vi "AIM664 Receive Data.vi"() -> ()   [LabVIEW 2020]
uses:
  src/AIM664LV.lvlib
panel:
  out "error out":errorcluster
  out "QueueIdOut 2":u32=664064
  out "GlobMonSize 2":u32=2153143691
  out "QueueIdOut":u32=664064
  out "GlobMonSize":u32=2153143691
  in  "Strobe":u32(ring) items=["FDX_MON_STROBE_DIS", "FDX_MON_STROBE_STOP", "FDX_MON_STROBE_START"]
  in  "TriggerPosition":u32
  in  "CaptureMode":u32(ring) items=["FDX_MON_SINGLE ", "FDX_MON_CONTINUOUS", "FDX_MON_SELECTIVE", "FDX_MON_RECORDING", "FDX_MON_REROS", "FDX_MON_HMU"]
  out "ResourceInfo 2":T1 {"PortMode" items=[" FDX_SINGLE", "FDX_REDUNDANT"]}
  out "ResourceInfo":T1 {"PortMode" items=[" FDX_SINGLE", "FDX_REDUNDANT"]}
  in  "Input Cluster 2":T2={"QueueCtrl"=1, "QueueId"=0, "RecordingFileName"="", "MaxFileSize"=0} {"QueueCtrl" items=["FDX_MON_QUEUE_CREATE", "FDX_MON_QUEUE_DELETE"]}
  in  "Stop":bool
  out "Output Cluste":T3={"EntryRead"=1, "BytesRead"=128, "Synchronized"=0, "ReadBuffer"=[192, 16, 128, 0, 192, 17, 128, 0, 0, 0, 0, 0, 0, 0, 0, 0, 60, 0, 0, 0, 64, 64, 0, 48, 84, 0, 128, 0, 104, 8, 0, 0, 33, 75, 42, 162, 3, 0, 0, 0, 0, 60, 2, 0, 0, 1, 33, 32, 8, 0, 69, 0, 0, 45, 0, 0, 64, 0, 1, 17, 109, 162, 10, 1, 33, 1, 224, 224, 0, 60, 0, 24, 0, 23, 0, 25, 0, 0, 65, 66, 67, 68, 69, 70, 71, 72, 73, 74, 75, 76, 77, 78, 79, 80, 81, 84, 0, 5, 0, 5, 0, 5, 0, 5, 0, 5, 0, 5, 0, 5, 0, 5, 0, 5, 0, 5, 0, 5, 0, 5, 0, 5, 0, 5, 0, 5, 0, 5, 0, 0, 0, 0, 0, 0, 0, 0, 0, 0, 0, 0, 0, 0, 0, 0, 0, 0, 0, 0, 0, 0, 0, 0, 0, 0, 0, 0, 0, 0, 0, 0, 0, 0, 0, 0, 0, 0, 0, 0, 0, 0, 0, 0, 0, 0, 0, 0, 0, 0, 0, 0, 0, 0, 0, 0, 0, 0, 0, 0, 0, 0, 0, 0, 0, 0, 0, 0, 0, 0, 0, 0, 0, 0, 0, 0, 0, 0, 0, 0, 0, 0, 0, 0, 0, 0, 0, 0, 0, 0, 0, 0, 0, 0, 0, 0, 0, 0, 0, 0, 0, 0, 0, 0, 0, 0, 0, 0, 0, 0, 0, 0, 0, 0, 0, 0, 0, 0, 0, 0, 0, 0, 0, 0, 0, 0, 0, 0, 0, 0, 0, 0, 0, 0, 0, 0, 0, 0, 0, 0, 0, 0, 0, 0, 0, 0, 0, 0, 0, 0, 0, 0, 0, 0, 0, 0, 0, 0, 0, 0, 0, 0, 0, 0, 0, 0, 0, 0, 0, 0, 0, 0, 0, 0, 0, 0, 0, 0, 0, 0, 0, 0, 0, 0, 0, 0, 0, 0, 0, 0, 0, 0, 0, 0, 0, 0, 0, 0, 0, 0, 0, 0, 0, 0, 0, 0, 0, 0, 0, 0, 0, 0, 0, 0, 0, 0, 0, 0, 0, 0, 0, 0, 0, 0, 0, 0, 0, 0, 0, 0, 0, 0, 0, 0, 0, 0, 0, 0, 0, 0, 0, 0, 0, 0, 0, 0, 0, 0, 0, 0, 0, 0, 0, 0, 0, 0, 0, 0, 0, 0, 0, 0, 0, 0, 0, 0, 0, 0, 0, 0, 0, 0, 0, 0, 0, 0, 0, 0, 0, 0, 0, 0, 0, 0, 0, 0, 0, 0, 0, 0, 0, 0, 0, 0, 0, 0, 0, 0, 0, 0, 0, 0, 0, 0, 0, 0, 0, 0, 0, 0, 0, 0, 0, 0, 0, 0, 0, 0, 0, 0, 0, 0, 0, 0, 0, 0, 0, 0, 0, 0, 0, 0, 0, 0, 0, 0, 0, 0, 0, 0, 0, 0, 0, 0, 0, 0, 0, 0, 0, 0, 0, 0, 0, 0, 0, 0, 0, 0, 0, 0, 0, 0, 0, 0, 0, 0, 0, 0, 0, 0, 0, 0, 0, 0, 0, 0, 0, 0, 0, 0, 0, 0, 0, 0, 0, 0, 0, 0, 0, 0, 0, 0, 0, 0, 0, 0, 0, 0, 0, 0, 0, 0, 0, 0, 0, 0, 0, 0, 0, 0, 0, 0, 0, 0, 0, 0, 0, 0, 0, 0, 0, 0, 0, 0, 0, 0, 0, 0, 0, 0, 0, 0, 0, 0, 0, 0, 0, 0, 0, 0, 0, 0, 0, 0, 0, 0, 0, 0, 0, 0, 0, 0, 0, 0, 0, 0, 0, 0, 0, 0, 0, 0, 0, 0, 0, 0, 0, 0, 0, 0, 0, 0, 0, 0, 0, 0, 0, 0, 0, 0, 0, 0, 0, 0, 0, 0, 0, 0, 0, 0, 0, 0, 0, 0, 0, 0, 0, 0, 0, 0, 0, 0, 0, 0, 0, 0, 0, 0, 0, 0, 0, 0, 0, 0, 0, 0, 0, 0, 0, 0, 0, 0, 0, 0, 0, 0, 0, 0, 0, 0, 0, 0, 0, 0, 0, 0, 0, 0, 0, 0, 0, 0, 0, 0, 0, 0, 0, 0, 0, 0, 0, 0, 0, 0, 0, 0, 0, 0, 0, 0, 0, 0, 0, 0, 0, 0, 0, 0, 0, 0, 0, 0, 0, 0, 0, 0, 0, 0, 0, 0, 0, 0, 0, 0, 0, 0, 0, 0, 0, 0, 0, 0, 0, 0, 0, 0, 0, 0, 0, 0, 0, 0, 0, 0, 0, 0, 0, 0, 0, 0, 0, 0, 0, 0, 0, 0, 0, 0, 0, 0, 0, 0, 0, 0, 0, 0, 0, 0, 0, 0, 0, 0, 0, 0, 0, 0, 0, 0, 0, 0, 0, 0, 0, 0, 0, 0, 0, 0, 0, 0, 0, 0, 0, 0, 0, 0, 0, 0, 0, 0, 0, 0, 0, 0, 0, 0, 0, 0, 0, 0, 0, 0, 0, 0, 0, 0, 0, 0, 0, 0, 0, 0, 0, 0, 0, 0, 0, 0, 0, 0, 0, 0, 0, 0, 0, 0, 0, 0, 0, 0, 0, 0, 0, 0, 0, 0, 0, 0, 0, 0, 0, 0, 0, 0, 0, 0, 0, 0, 0, 0, 0, 0, 0, 0, 0, 0, 0, 0, 0, 0, 0, 0, 0, 0, 0, 0, 0, 0, 0, 0, 0, 0, 0, 0, 0, 0, 0, 0, 0, 0, 0, 0, 0, 0, 0, 0, 0, 0, 0, 0, 0, 0, 0, 0, 0, 0, 0, 0, 0, 0, 0, 0, 0, 0, 0, 0, 0, 0, 0, 0, 0, 0, 0, 0, 0, 0, 0, 0, 0, 0, 0, 0, 0, 0, 0, 0, 0, 0, 0, 0, 0, 0, 0, 0, 0, 0, 0, 0, 0, 0, 0, 0, 0, 0, 0, 0, 0, 0, 0, 0, 0, 0, 0, 0, 0, 0, 0, 0, 0, 0, 0, 0, 0, 0, 0, 0, 0, 0, 0, 0, 0, 0, 0, 0, 0, 0, 0, 0, 0, 0, 0, 0, 0, 0, 0, 0, 0, 0, 0, 0, 0, 0, 0, 0, 0, 0, 0, 0, 0, 0, 0, 0, 0, 0, 0, 0, 0, 0, 0, 0, 0, 0, 0, 0, 0, 0, 0, 0, 0, 0, 0, 0, 0, 0, 0, 0, 0, 0, 0, 0, 0, 0, 0, 0, 0, 0, 0, 0, 0, 0, 0, 0, 0, 0, 0, 0, 0, 0, 0, 0, 0, 0, 0, 0, 0, 0, 0, 0, 0, 0, 0, 0, 0, 0, 0, 0, 0, 0, 0, 0, 0, 0, 0, 0, 0, 0, 0, 0, 0, 0, 0, 0, 0, 0, 0, 0, 0, 0, 0, 0, 0, 0, 0, 0, 0, 0, 0, 0, 0, 0, 0, 0, 0, 0, 0, 0, 0, 0, 0, 0, 0, 0, 0, 0, 0, 0, 0, 0, 0, 0, 0, 0, 0, 0, 0, 0, 0, 0, 0, 0, 0, 0, 0, 0, 0, 0, 0, 0, 0, 0, 0, 0, 0, 0, 0, 0, 0, 0, 0, 0, 0, 0, 0, 0, 0, 0, 0, 0, 0, 0, 0, 0, 0, 0, 0, 0, 0, 0, 0, 0, 0, 0, 0, 0, 0, 0, 0, 0, 0, 0, 0, 0, 0, 0, 0, 0, 0, 0, 0, 0, 0, 0, 0, 0, 0, 0, 0, 0, 0, 0, 0, 0, 0, 0, 0, 0, 0, 0, 0, 0, 0, 0, 0, 0, 0, 0, 0, 0, 0, 0, 0, 0, 0, 0, 0, 0, 0, 0, 0, 0, 0, 0, 0, 0, 0, 0, 0, 0, 0, 0, 0, 0, 0, 0, 0, 0, 0, 0, 0, 0, 0, 0, 0, 0, 0, 0, 0, 0, 0, 0, 0, 0, 0, 0, 0, 0, 0, 0, 0, 0, 0, 0, 0, 0, 0, 0, 0, 0, 0, 0, 0, 0, 0, 0, 0, 0, 0, 0, 0, 0, 0, 0, 0, 0, 0, 0, 0, 0, 0, 0, 0, 0, 0, 0, 0, 0, 0, 0, 0, 0, 0, 0, 0, 0, 0, 0, 0, 0, 0, 0, 0, 0, 0, 0, 0, 0, 0, 0, 0, 0, 0, 0, 0, 0, 0, 0, 0, 0, 0, 0, 0, 0, 0, 0, 0, 0, 0, 0, 0, 0, 0, 0, 0, 0, 0, 0, 0, 0, 0, 0, 0, 0, 0, 0, 0, 0, 0, 0, 0, 0, 0, 0, 0, 0, 0, 0, 0, 0, 0, 0, 0, 0, 0, 0, 0, 0, 0, 0, 0, 0, 0, 0, 0, 0, 0, 0, 0, 0, 0, 0, 0, 0, 0, 0, 0, 0, 0, 0, 0, 0, 0, 0, 0, 0, 0, 0, 0, 0, 0, 0, 0, 0, 0, 0, 0, 0, 0, 0, 0, 0, 0, 0, 0, 0, 0, 0, 0, 0, 0, 0, 0, 0, 0, 0, 0, 0, 0, 0, 0, 0, 0, 0, 0, 0, 0, 0, 0, 0, 0, 0, 0, 0, 0, 0, 0, 0, 0, 0, 0, 0, 0, 0, 0, 0, 0, 0, 0, 0, 0, 0, 0, 0, 0, 0, 0, 0, 0, 0, 0, 0, 0, 0, 0, 0, 0, 0, 0, 0, 0, 0, 0, 0, 0, 0, 0, 0, 0, 0, 0, 0, 0, 0, 0, 0, 0, 0, 0, 0, 0, 0, 0, 0, 0, 0, 0, 0, 0, 0, 0, 0, 0, 0, 0, 0, 0, 0, 0, 0, 0, 0, 0, 0, 0, 0, 0, 0, 0, 0, 0, 0, 0, 0, 0, 0, 0, 0, 0, 0, 0, 0, 0, 0, 0, 0, 0, 0, 0, 0, 0, 0, 0, 0, 0, 0, 0, 0, 0, 0, 0, 0, 0, 0, 0, 0, 0, 0, 0, 0, 0, 0, 0, 0, 0, 0, 0, 0, 0, 0, 0, 0, 0, 0]} {"ReadBuffer" format="%x"}
  in  "Input Cluster":T4={"QueueId"=0, "EntryCount"=1, "ReadQualifier"=0, "MaxReadBytes"=1600} {"ReadQualifier" items=["FDX_MON_READ_FULL", "FDX_MON_READ_HEADER", "FDX_MON_READ_DATA"]}
  out "Output Cluster":T5={"MonStatus"=2, "FramesCaptured"=532, "BytesRecordedHiPart"=16779328, "BytesRecordedLoPart"=50331632} {"MonStatus" items=["FDX_MON_OFF", "FDX_MON_WAIT_FOR_TRIGGER", "FDX_MON_TRIGGERED", "FDX_MON_STOPPED", "FDX_MON_FULL"]}
  in  "Input Cluster":T2 {"QueueCtrl" items=["FDX_MON_QUEUE_CREATE", "FDX_MON_QUEUE_DELETE"]}
  in  "Input Cluster":T6={"ReceiveMode"=0, "DefaultPayloadMode"=0, "DefaultCronoMode"=1, "GlbMonBufferSizeIn"=0, "RerosDefaultOutputPortmap"=0} {"DefaultCronoMode" items=["cFDX_RX_DEFAULT_ENA_CNT", "FDX_RX_DEFAULT_MON_ENA_ALL", "FDX_RX_DEFAULT_MON_ENA_GOOD"]; "DefaultPayloadMode" items=["FDX_PAYLOAD_FULL", "FDX_PAYLOAD_IP_EXT", "FDX_PAYLOAD_IP", "FDX_PAYLOAD_MAC"]; "ReceiveMode" items=["FDX_RX_CHRONO", "FDX_RX_VL"]}
  out "GlbMonBufferSizeOut":u32=16777216
  in  "Input Cluster":T7={"SrvName"="local", "ClHostName"="local", "ClUser"="Brett", "ClApplication"="Test", "ClApplicationVersion"="V01.00", "ResourceID"=2, "Privileges"=4294967295} {"Privileges" items=["PRIVILEGES_ADMIN"=4294967295]}
  in  "Input Cluster":T7={"SrvName"="local", "ClHostName"="local", "ClUser"="Brett", "ClApplication"="Test", "ClApplicationVersion"="V01.00", "ResourceID"=1, "Privileges"=4294967295} {"Privileges" items=["PRIVILEGES_ADMIN"=4294967295]}
  in  "Input Cluster":T8={"SrvName"="local", "ResourceID"=1, "ResourceType"=0} {"ResourceType" items=["Board", "Port"]}
  out "Output Cluster 2":T9={"ResourceID"=1, "ResourceType"=0, "ResourceInfo"="AMC-FDX-2", "StructId"=0}
  in  "ServerRElement":u32=1
  in  "Input Cluster":T8={"SrvName"="local", "ResourceID"=2, "ResourceType"=1} {"ResourceType" items=["Board", "Port"]}
  out "Output Cluster":T9={"ResourceID"=2, "ResourceType"=1, "ResourceInfo"="Port1", "StructId"=0}
  in  "ServerRElement":u32=2
  out "NuOfResources":u32=3
  in  "SrvName":string="local"
  out "NuOfServers":u32=1
  # "ARINC 664 Receive Data"
  # "Overview: Configure the board to Receive Data.\nRequirement: At least one AIM ARINC-664 board with installed AIM ARINC 664 BSP.\nRestrictions: None.\nInstruction:\n1. Run the VI.\n2. Verify the results in the indicators."
  # "Rx Port"
  # "Board"
  # "Rx Port"
  # "Board"
  # "FdxInitCvi"
  # "FdxLogoutCvi"
  # "CountServerResourcesCvi"
  # "GetServerResourcesCvi"
  # "QueryServerResourceCvi"
  # "FdxLoginCvi"
  # "FdxLogoutCvi"
  # "GetServerResourcesCvi"
  # "QueryServerResourceCvi"
  # "FdxRxModeControlCvi"
  # "FdxRxMonCaptureControlCvi"
  # "FdxLoginCvi"
  # "FdxCmdMonQueueControl"
  # "FdxRxControlCvi"
  # "FdxCmdMonQueueControl"
  # "FdxMonGetStatusCvii"
  # "FdxRxControlCvi"
  # "FdxCmdMonQueueReadCvii"
  # "Input"
  # "Input"
  # "Input"
  # "Input"
  # "Input"
  # "Input"
  # "Input"
  # "Input"
  # "Output"
  # "Input"
  # "Input"
  # "Input"
  # "Input"
  # "Input"
  # "Input"
  # "Input"
  # "Output"
  # "Output"
  # "Output"
  # "Output"
  # "Output"
  # "Output"
  # "Output"
  # "Output"
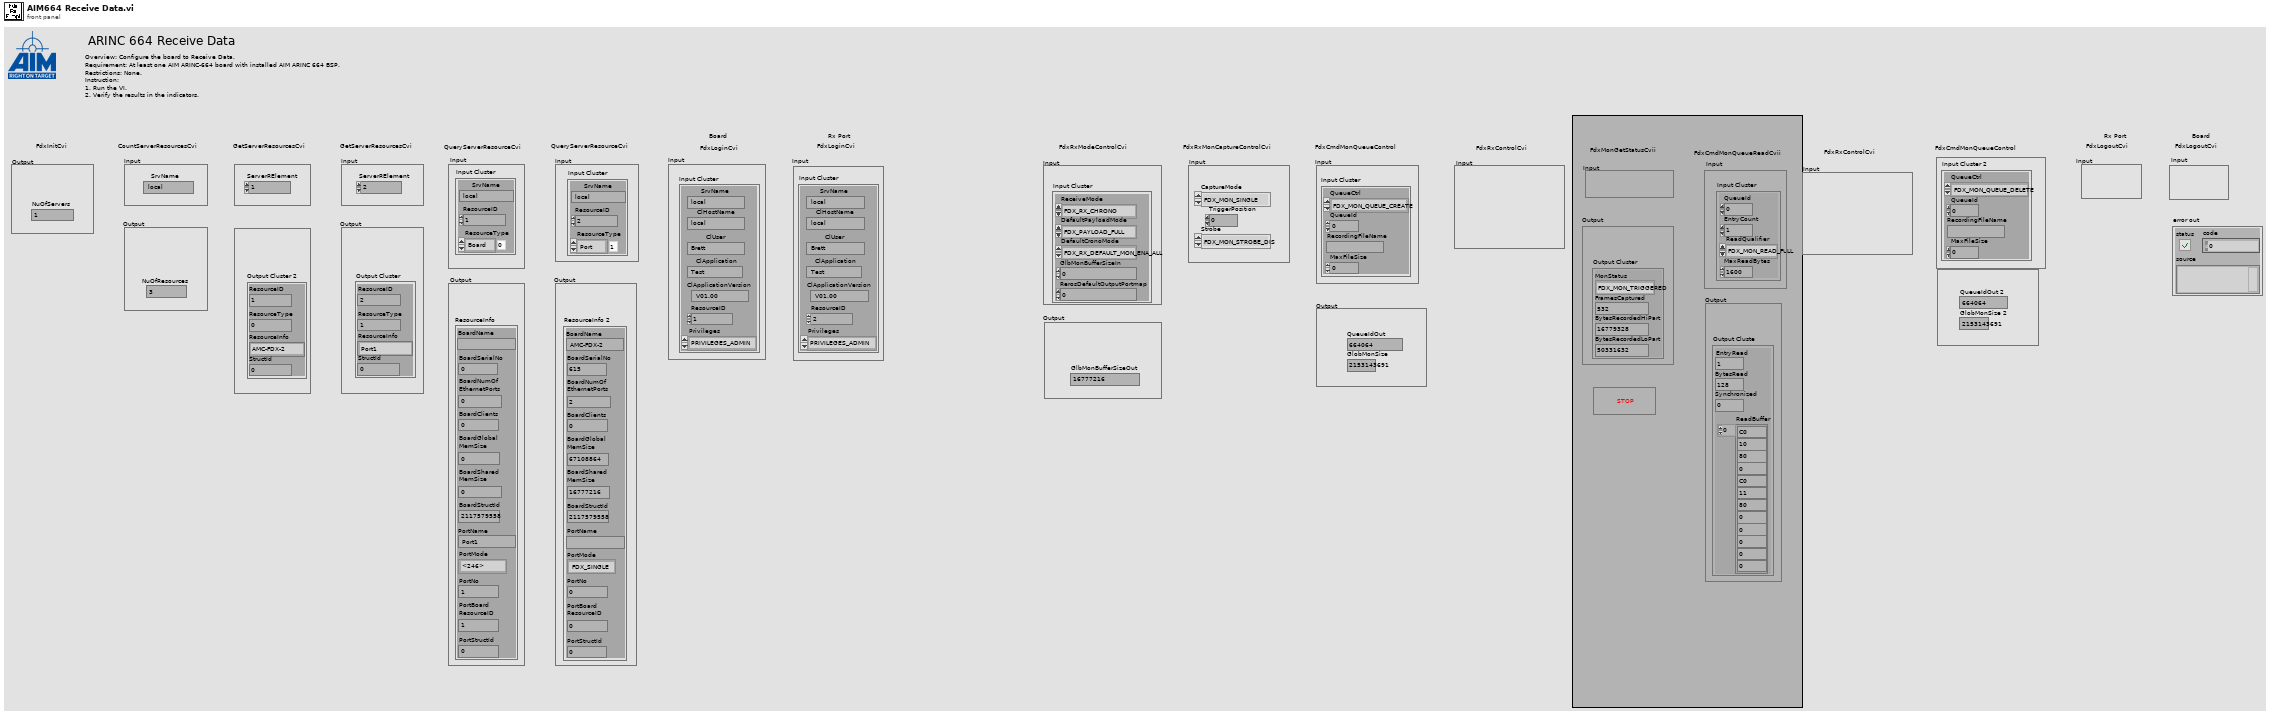
[diagram p1: front panel]
types:
  T1 = cluster{"BoardName":string, "BoardSerialNo":u32, "BoardNumOf\nEthernetPorts":u32, "BoardClients":u32, "BoardGlobal\nMemSize":u32, "BoardShared\nMemSize":u32, "BoardStructId":u32, "PortName":string, "PortMode":u32, "PortNo":u32, "PortBoard\nResourceID":u32, "PortStructId":u32}
  T2 = cluster{"QueueCtrl":u32, "QueueId":u32, "RecordingFileName":string, "MaxFileSize":u32}
  T3 = cluster{"EntryRead":u32, "BytesRead":u32, "Synchronized":u32, "ReadBuffer":u8[]}
  T4 = cluster{"QueueId":u32, "EntryCount":u32, "ReadQualifier":u32, "MaxReadBytes":u32}
  T5 = cluster{"MonStatus":u32, "FramesCaptured":u32, "BytesRecordedHiPart":u32, "BytesRecordedLoPart":u32}
  T6 = cluster{"ReceiveMode":u32, "DefaultPayloadMode":u32, "DefaultCronoMode":u32, "GlbMonBufferSizeIn":u32, "RerosDefaultOutputPortmap":u32}
  T7 = cluster{"SrvName":string, "ClHostName":string, "ClUser":string, "ClApplication":string, "ClApplicationVersion":string, "ResourceID":u32, "Privileges":u32}
  T8 = cluster{"SrvName":string, "ResourceID":u32, "ResourceType":u32}
  T9 = cluster{"ResourceID":u32, "ResourceType":u32, "ResourceInfo":string, "StructId":u32}
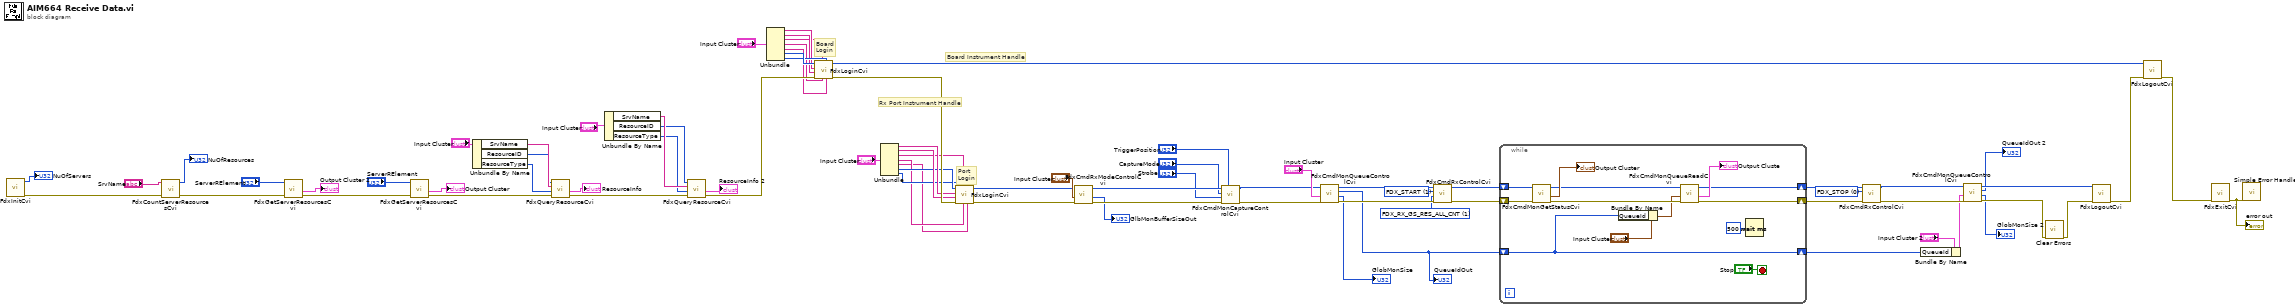
[diagram p0: block diagram]
diagram:
  w9 = u32 1 items=["FDX_RX_GS_RES_NO_CNT", "FDX_RX_GS_RES_ALL_CNT", "FDX_RX_GS_RES_ERR_CNT "] ("GlobalStatisticReset")
  w10 = u32 1 items=["FDX_STOP", "FDX_START"] ("StartMode")
  w11 = u32 0 items=["FDX_STOP", "FDX_START"] ("StartMode")
  # "Rx Port Instrument Handle"
  # "Port\nLogin"
  # "Board Instrument Handle"
  # "Board\nLogin"
  n1 = call "FdxInitCvi.vi"() -> ("error out"=w76:errorcluster, "Number of Servers"=→"NuOfServers":u32)  [unwired: 10 in]
  n2 = call "FdxCountServerResourcesCvi.vi"("error in"=w76, "SrvName (local)"="SrvName") -> ("error out"=w75:errorcluster, "Number of Resources"=→"NuOfResources":u32)  [unwired: 8 in]
  n3 = call "FdxGetServerResourcesCvi.vi"("error in"=w75, "ServerRElement"="ServerRElement") -> ("error out"=w74:errorcluster, "ServerResourceInfo"=→"Output Cluster 2":T9)  [unwired: 4 in, 4 out]
  n4 = call "FdxGetServerResourcesCvi.vi"("error in"=w74, "ServerRElement"="ServerRElement") -> ("error out"=w77:errorcluster, "ServerResourceInfo"=→"Output Cluster":T9)  [unwired: 4 in, 4 out]
  n5 = Unbundle By Name("Input Cluster") -> ("SrvName"=w45:string, "ResourceID"=w44:u32, "ResourceType"=w43:u32)
  n6 = call "FdxQueryResourceCvi.vi"("error in"=w77, "ResourceType"=w43, "SrvName"=w45, "ResourceID"=w44) -> ("error out"=w73:errorcluster, "ResourceInfo"=→"ResourceInfo":T1)  [unwired: 5 in, 1 out]
  n7 = Unbundle By Name("Input Cluster") -> ("SrvName"=w41:string, "ResourceID"=w40:u32, "ResourceType"=w39:u32)
  n8 = call "FdxQueryResourceCvi.vi"("error in"=w73, "ResourceType"=w39, "SrvName"=w41, "ResourceID"=w40) -> ("error out"=w72:errorcluster, "ResourceInfo"=→"ResourceInfo 2":T1)  [unwired: 5 in, 1 out]
  n9 = Unbundle("Input Cluster") -> ("SrvName"=w35:string, "ClHostName"=w34:string, "ClUser"=w33:string, "ClApplication"=w32:string, "ClApplicationVersion"=w31:string, "ResourceID"=w37:u32, "Privileges"=w36:u32)
  n10 = call "FdxLoginCvi.vi"("ClApplicationVersion"=w31, "Privileges"=w36, "ClApplication"=w32, "ClUser"=w33, "error in"=w72, "ClHostName"=w34, "SrvName"=w35, "ResourceID"=w37) -> ("error out"=w67:errorcluster, "InstrumentHandle"=w58:u32)  [unwired: 2 in]
  n11 = Unbundle("Input Cluster") -> ("SrvName"=w29:string, "ClHostName"=w28:string, "ClUser"=w25:string, "ClApplication"=w24:string, "ClApplicationVersion"=w23:string, "ResourceID"=w27:u32, "Privileges"=w26:u32)
  n12 = call "FdxLoginCvi.vi"("ClApplicationVersion"=w23, "Privileges"=w26, "ClApplication"=w24, "ClUser"=w25, "error in"=w67, "ClHostName"=w28, "SrvName"=w29, "ResourceID"=w27) -> ("error out"=w66:errorcluster, "InstrumentHandle"=w22:u32)  [unwired: 2 in]
  n13 = call "FdxCmdRxModeControlCvi.vi"("error in"=w66, "RxModeControlIn"="Input Cluster", "InstrumentHandle_port"=w22) -> ("error out"=w71:errorcluster, "GlbMonBufferSizeOut"=→"GlbMonBufferSizeOut":u32, "InstrumentHandle_port"=w21:u32)  [unwired: 6 in]
  n14 = call "FdxCmdMonCaptureControlCvi.vi"("TriggerPosition"="TriggerPosition", "error in"=w71, "Strobe"="Strobe", "CaptureMode"="CaptureMode", "InstrumentHandle_port"=w21) -> ("error out"=w70:errorcluster, "InstrumentHandle_port"=w20:u32)  [unwired: 5 in]
  n15 = call "FdxCmdMonQueueControlCvi.vi"("error in"=w70, "Q Ctrl In"="Input Cluster", "InstrumentHandle_port"=w20) -> ("error out"=w69:errorcluster, "GlobMonSize"=→"GlobMonSize":u32, "QueueIdOut"=w5:u32, "InstrumentHandle_port"=w19:u32)  [unwired: 5 in]
  "QueueIdOut" <- w5
  n16 = call "FdxCmdRxControlCvi.vi"("error in"=w69, "GlobalStatisticReset"=w9, "StartMode"=w10, "InstrumentHandle_port"=w19) -> ("error out"=w65:errorcluster, "InstrumentHandle_port"=w18:u32)  [unwired: 6 in]
  n17 = while {
    shift-right: [w78] -> w17
    shift-left: w18 -> [w81]
    shift-right: [w80] -> w14
    shift-left: w65 -> [w89]
    shift-right: [w82] -> w51
    shift-left: w5 -> [w82]
    stop <- "Stop" stop-if-true
    n18 = call "FdxCmdMonGetStatusCvi.vi"("error in"=w89, "InstrumentHandle_port"=w81) -> ("error out"=w90:errorcluster, "MonStatus"=→"Output Cluster":T5, "InstrumentHandle_port"=w79:u32)  [unwired: 7 in]
    n19 = Bundle By Name(cluster="Input Cluster", "QueueId"=w82) -> (w86:T4)
    n20 = call "FdxCmdMonQueueReadCvi.vi"("error in"=w90, "QueueReadIn"=w86, "InstrumentHandle_port"=w79) -> ("error out"=w80:errorcluster, "QueueReadOut"=→"Output Cluste":T3, "InstrumentHandle_port"=w78:u32)  [unwired: 6 in]
    n21 = Wait (ms)(milliseconds to wait=u32 500 ("Zu wartende ms")) -> ()  [unwired: 1 out]
  }
  n22 = call "FdxCmdRxControlCvi.vi"("error in"=w14, "StartMode"=w11, "InstrumentHandle_port"=w17) -> ("error out"=w64:errorcluster, "InstrumentHandle_port"=w16:u32)  [unwired: 7 in]
  n23 = Bundle By Name(cluster="Input Cluster 2", "QueueId"=w51) -> (w52:T2)
  n24 = call "FdxCmdMonQueueControlCvi.vi"("error in"=w64, "Q Ctrl In"=w52, "InstrumentHandle_port"=w16) -> ("error out"=w13:errorcluster, "GlobMonSize"=→"GlobMonSize 2":u32, "QueueIdOut"=→"QueueIdOut 2":u32, "InstrumentHandle_port"=w15:u32)  [unwired: 5 in]
  n25 = call <vilib>:"Clear Errors.vi"("error in (no error)"=w13) -> ("error out"=w12:errorcluster)  [unwired: 5 in, 1 out]
  n26 = call "FdxLogoutCvi.vi"("error in"=w12, "InstrumentHandle"=w15) -> ("error out"=w68:errorcluster)  [unwired: 9 in]
  n27 = call "FdxLogoutCvi.vi"("error in"=w68, "InstrumentHandle"=w58) -> ("error out"=w63:errorcluster)  [unwired: 9 in]
  n28 = call "FdxExitCvi.vi"("error in"=w63) -> ("error out"=w1:errorcluster)  [unwired: 10 in]
  "error out" <- w1
  n29 = call <vilib>:"Simple Error Handler.vi"("error in (no error)"=w1) -> ()  [unwired: 4 in, 5 out]
